vi "data_retrieval_processing_sequence.vi"() -> ()   [LabVIEW 2021]
uses:
  a5b8f340-0aaf-3fc0-001e-aaef3e36ac3f.vi
  1634fdf6-5eff-3fe9-09cf-f9bccf8fe73f.vi
panel:
  out "time spent (ms)":u32
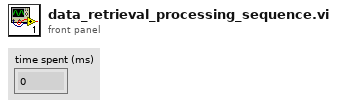
[diagram p1: front panel]
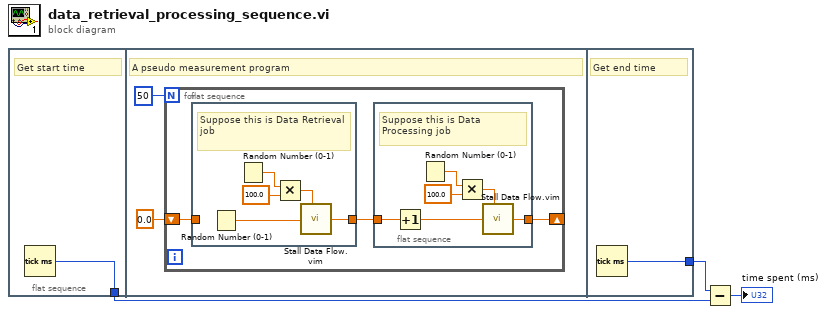
[diagram p0: block diagram]
diagram:
  n1 = flat-sequence {
    tunnel: [w4] -> w2
    tunnel: [w21] -> w3
    frame #0 {
      # "Get start time"
      n2 = Tick Count (ms)() -> (millisecond timer value=w4:u32)
    }
    frame #1 {
      # "A pseudo measurement program"
      n3 = for {
        N: 50 -> [_]
        shift-right: [w7] -> _
        shift-left: 0.0 -> [w9]
        n4 = flat-sequence {
          tunnel: w9 -> [_]
          tunnel: [w20] -> w8
          frame #0 {
            # "Suppose this is Data Retrieval job"
            n5 = Random Number (0-1)() -> (number: 0 to 1=w16:dbl)
            n6 = Random Number (0-1)() -> (number: 0 to 1=w19:dbl)
            n7 = Multiply(x=w19, y=100.0) -> (x*y=w17:dbl)
            n8 = call "Stall Data Flow.vim"("value in"=w16, "milliseconds to wait"=w17) -> ("value out"=w20:dbl)  [unwired: 1 out]
          }
        }
        n9 = flat-sequence {
          tunnel: w8 -> [w11]
          tunnel: [w15] -> w7
          frame #0 {
            # "Suppose this is Data Processing job"
            n10 = Increment(x=w11) -> (x+1=w10:dbl)
            n11 = Random Number (0-1)() -> (number: 0 to 1=w13:dbl)
            n12 = Multiply(x=w13, y=100.0) -> (x*y=w12:dbl)
            n13 = call "Stall Data Flow.vim"("value in"=w10, "milliseconds to wait"=w12) -> ("value out"=w15:dbl)  [unwired: 1 out]
          }
        }
      }
    }
    frame #2 {
      # "Get end time"
      n14 = Tick Count (ms)() -> (millisecond timer value=w21:u32)
    }
  }
  n15 = Subtract(x=w3, y=w2) -> (x-y=→"time spent (ms)":u32)
